vi "Actor Core.vi"(8 "error in":errorcluster, 11 "Measure Object in":refnum<class "Stepper.lvclass">) -> (0 "error out":errorcluster, 3 "Actor out":refnum<class "Actor.lvclass">)   [LabVIEW 2021, in "Stepper.lvclass"]
doc: "(<B>Filename</B>: Actor Framework.lvlib:Actor.lvclass:Actor Core.vi)\n\nReceives messages to the actor, reacts to them, and initiates any error handling that may shut the actor down.\n\nDescendant classes may override this VI to append parallel tasks for the actor to complete while it handles messages. Overrides use the Call Parent Method node."
uses:
  Stepper.lvclass
  Continuous Recorder Actor/Continuous Recorder Actor.lvclass
  <vilib>/ActorFramework/Actor/Actor.lvclass
  NHMFL_Core/Libraries/Instruments/Controls/Stepper Config.ctl
panel:
  in  "Configuration":T1={"Start"=-0.001, "End"=0.001, "Step"=0.0001, "Append measurements"=[]} {"Step" format="%#_6p"; "End" format="%#_6p"; "Start" format="%#_6p"}
  out "Name":string
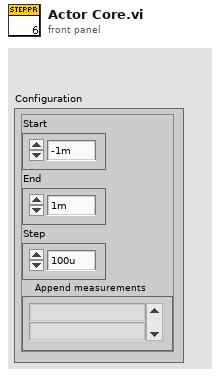
[diagram p1: front panel]
types:
  T1 = typedef "Stepper Config.ctl" = cluster{"Start":dbl, "End":dbl, "Step":dbl, "Append measurements":string[]}
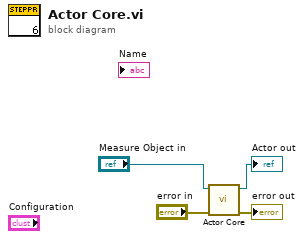
[diagram p0: block diagram]
diagram:
  n1 = call-parent "Actor Core.vi"("error in"="error in", "Measure Object in"="Measure Object in") -> ("error out"=→"error out":errorcluster, "Actor out"=→"Actor out":refnum<class "Actor.lvclass">)  [unwired: 8 in]
